vi "Controller Write Boolean.vi"(8 "Error In":errorcluster, 10 "Values":bool[](array[boolean]), 11 "Variables":refnum<k21>[](array[refnum])) -> (0 "Error Out":errorcluster)   [LabVIEW 2011, in "Controller VIs.lvlib"]
doc: "Writes a vector of fixed-Point <+/-,20,5> I/O variables."
uses:
  Controller VIs.lvlib
panel:
  out "a":refnum<k21>
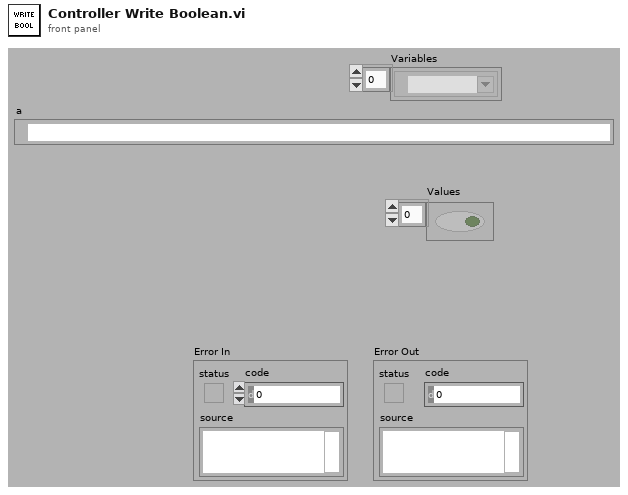
[diagram p1: front panel]
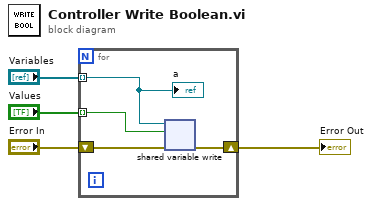
[diagram p0: block diagram]
diagram:
  n1 = for {
    tunnel: "Values" -> [w8] mode=indexing
    tunnel: "Variables" -> [w5] mode=indexing
    shift-right: [w6] -> w3
    shift-left: "Error In" -> [w7]
    n2 = shared-variable-write(w5, w7, w8) -> (w6:errorcluster)  [unwired: 1 out]
    "a" <- w5
  }
  "Error Out" <- w3
